vi "Initialize.vi"(7 "Release all channels first":bool=TRUE, 8 "error in (no error)":errorcluster, 9 "TPCANBaudrate":T1, 10 "Channel(1~6)":u8=1, 11 "PCANUSB in":refnum<class "PCANUSB.lvclass">) -> (0 "error out":errorcluster, 3 "PCANUSB out":refnum<class "PCANUSB.lvclass">)   [LabVIEW 2024, in "PCANUSB.lvclass"]
uses:
  PCANUSB.lvclass
  PCAN/CAN Communication.llb/TPCANBaudrate.ctl
  PCAN/CAN Communication.llb/TPCANParameter.ctl
  PCAN/API_for_PCAN_BASIC_FD/TPCANHandle.ctl
  PCANUSB.lvclass/PCANUSB.ctl
  PCAN/CAN Communication.llb/PCAN Get CHANNEL CONDITION.vi
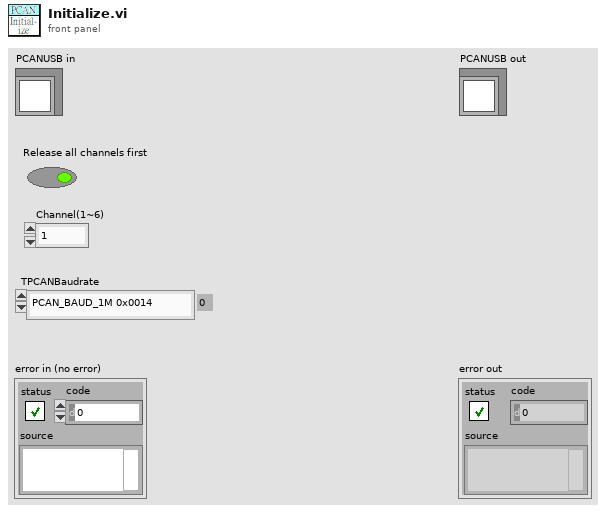
[diagram p1: front panel]
types:
  T1 = typedef "TPCANBaudrate.ctl" = enum16{"PCAN_BAUD_1M 0x0014", "PCAN_BAUD_800K 0x0016", "PCAN_BAUD_500K 0x001C", "PCAN_BAUD_250K 0x011C", "PCAN_BAUD_125K 0x031C", "PCAN_BAUD_100K 0x432F", "PCAN_BAUD_95K 0xC34E", "PCAN_BAUD_83K 0x852B", "PCAN_BAUD_50K 0x472F", "PCAN_BAUD_47K 0x1414", "PCAN_BAUD_33K 0x8B2F", "PCAN_BAUD_20K 0x532F", "PCAN_BAUD_10K 0x672F", "PCAN_BAUD_5K 0x7F7F", "User Baudrate"}
  T2 = typedef "TPCANParameter.ctl" = enum8{"Not Available", "PCAN device number", "PCAN 5-volt power", "PCAN receive event", "PCAN message filter", "PCAN API version", "PCAN channel version", "PCAN busoff autoreset", "PCAN listen-only", "PCAN log location", "PCAN log status", "PCAN log configure", "PCAN log text", "PCAN channel condition", "PCAN hardware name", "PCAN_RECEIVE_STATUS", "PCAN_CONTROLLER_NUMBER", "PCAN_TRACE_LOCATION ", "PCAN_TRACE_STATUS", "PCAN_TRACE_SIZE", "PCAN_TRACE_CONFIGURE", "PCAN_CHANNEL_IDENTIFYING", "PCAN_CHANNEL_FEATURES", "PCAN_SPEED_ADAPTING", "PCAN_BITRATE_INFO", "PCAN_BITRATE_INFO_FD", "PCAN_BUSSPEED_NOMINAL", "PCAN_BUSSPEED_DATA", "PCAN_IP_ADDRESS", "PCAN_LAN_SERVICE_STATUS", "PCAN_ALLOW_STATUS_FRAMES", "PCAN_ALLOW_RTR_FRAMES", "PCAN_ALLOW_ERROR_FRAMES", "PCAN_INTERFRAME_DELAY", "PCAN_ACCEPTANCE_FILTER_11BIT", "PCAN_ACCEPTANCE_FILTER_29BIT", "PCAN_IO_DIGITAL_CONFIGURATION", "PCAN_IO_DIGITAL_VALUE", "PCAN_IO_DIGITAL_SET", "PCAN_IO_DIGITAL_CLEAR", "PCAN_IO_ANALOG_VALUE"}
  T3 = typedef "TPCANHandle.ctl" = enum16{"PCAN_NONEBUS  0x000", "PCAN_ISABUS1  0x21", "PCAN_ISABUS2  0x22", "PCAN_ISABUS3  0x23", "PCAN_ISABUS4  0x24", "PCAN_ISABUS5  0x25", "PCAN_ISABUS6  0x26", "PCAN_ISABUS7  0x27", "PCAN_ISABUS8  0x28", "PCAN_DNGBUS1  0x31", "PCAN_PCIBUS1  0x41", "PCAN_PCIBUS1  0x42", "PCAN_PCIBUS1  0x43", "PCAN_PCIBUS1  0x44", "PCAN_PCIBUS1  0x45", "PCAN_PCIBUS1  0x46", "PCAN_PCIBUS1  0x47", "PCAN_PCIBUS1  0x48", "PCAN_PCIBUS1  0x409", "PCAN_PCIBUS1  0x40A", "PCAN_PCIBUS1  0x40B", "PCAN_PCIBUS1  0x40C", "PCAN_PCIBUS1  0x40D", "PCAN_PCIBUS1  0x40E", "PCAN_PCIBUS1  0x40F", "PCAN_PCIBUS1  0x410", "PCAN_USBBUS1  0x51", "PCAN_USBBUS2  0x52", "PCAN_USBBUS3  0x53", "PCAN_USBBUS4  0x54", "PCAN_USBBUS5  0x55", "PCAN_USBBUS6  0x56", "PCAN_USBBUS7  0x57", "PCAN_USBBUS8  0x58", "PCAN_USBBUS9  0x509", "PCAN_USBBUS10  0x50A", "PCAN_USBBUS11  0x50B", "PCAN_USBBUS12  0x50C", "PCAN_USBBUS13  0x50D", "PCAN_USBBUS14  0x50E", "PCAN_USBBUS15  0x50F", "PCAN_USBBUS16  0x510", "PCAN_PCCBUS1  0x61", "PCAN_PCCBUS2  0x62", "PCAN_LANBUS1  0x801", "PCAN_LANBUS2  0x802", "PCAN_LANBUS3  0x803", "PCAN_LANBUS4  0x804", "PCAN_LANBUS5  0x805", "PCAN_LANBUS6  0x806", "PCAN_LANBUS7  0x807", "PCAN_LANBUS8  0x808", "PCAN_LANBUS9  0x809", "PCAN_LANBUS10  0x80A", "PCAN_LANBUS11  0x80B", "PCAN_LANBUS12  0x80C", "PCAN_LANBUS13  0x80D", "PCAN_LANBUS14  0x80E", "PCAN_LANBUS15  0x80F", "PCAN_LANBUS16  0x810"}
  T4 = typedef "Channel Availability.ctl" = enum16{"PCAN_CHANNEL_UNAVAILABLE", "PCAN_CHANNEL_AVAILABLE", "PCAN_CHANNEL_OCCUPIED"}
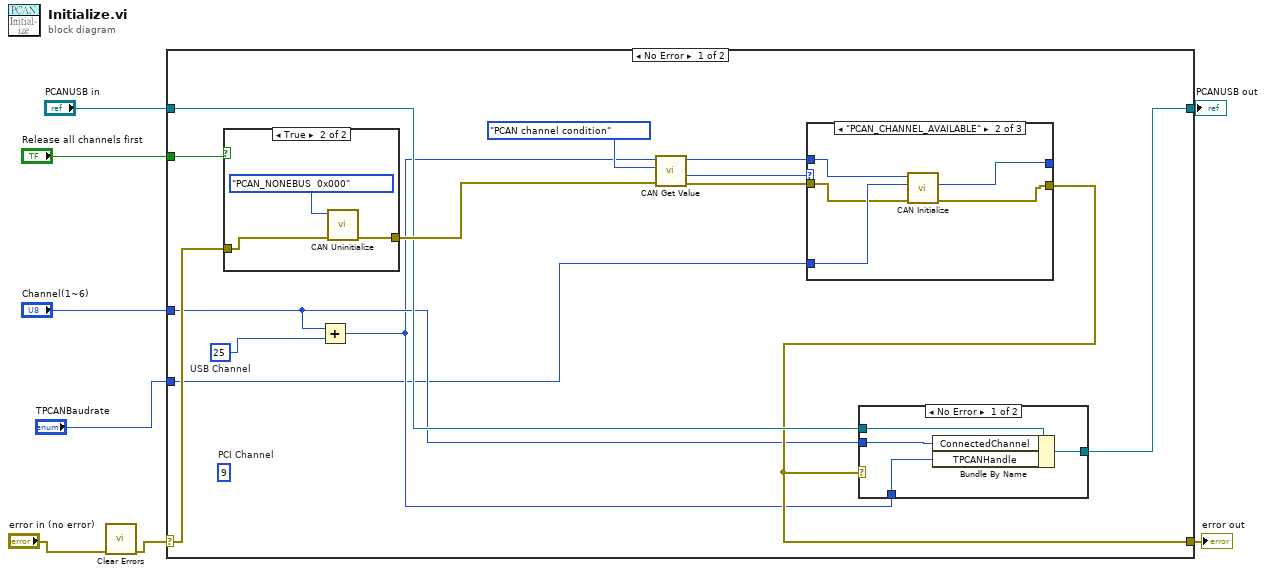
[diagram p0: block diagram]
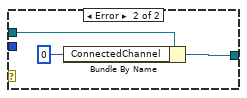
[diagram p2: hidden frame]
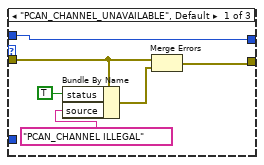
[diagram p3: hidden frame]
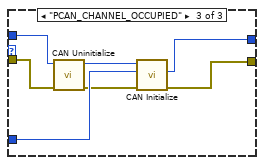
[diagram p4: hidden frame]
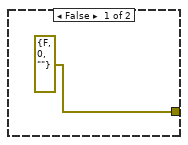
[diagram p5: hidden frame]
diagram:
  n1 = call <vilib>:"Clear Errors.vi"("error in (no error)"="error in (no error)") -> ("error out"=w1:errorcluster)  [unwired: 5 in, 1 out]
  n2 = case shown="No Error" w1 {
    selector: w1 -> [w21 w53]
    tunnel: [w13 w53] -> w8
    tunnel: [w14 w52] -> w6
    tunnel: "PCANUSB in" -> [w15 w52]
    tunnel: "Release all channels first" -> [w22 _]
    tunnel: "TPCANBaudrate" -> [w10 _]
    tunnel: "Channel(1~6)" -> [w12 _]
    frame No Error {
      w9 = 25  # USB Channel
      (unwired) 9  # PCI Channel
      n3 = case shown="True" w22 {
        tunnel: w21 -> [_ w50]
        tunnel: [errorcluster {"status"=FALSE, "code"=0, "source"=""} ("error constant") w49] -> w19
        frame False {
        }
        frame True {
          n4 = call "CAN Uninitialize.vi"("error in (no error)"=w50, "TPCANHandle"=TPCANHandle."PCAN_NONEBUS  0x000") -> ("error out"=w49:errorcluster)  [unwired: 7 in, 2 out]
        }
      }
      n5 = Add(x=w12, y=w9) -> (x+y=w11:i32)
      n6 = call-poly "CAN Get Value.vi"("error in (no error)"=w19, "TPCANParameter"=TPCANParameter."PCAN channel condition", "TPCANHandle"=w11) -> ("error out"=w17:errorcluster, "Channel condition"=w18:T4, "TPCANHandle out"=w16:T3)  [unwired: 6 in]
      n7 = case shown="\"PCAN_CHANNEL_AVAILABLE\"" w18 {
        tunnel: w17 -> [w33 w36 w47]
        tunnel: [w31 w37 w41] -> w13
        tunnel: w16 -> [w30 w40 w46]
        tunnel: w10 -> [_ w39 w44]
        tunnel: [w30 w38 w42] -> _
        frame "PCAN_CHANNEL_UNAVAILABLE", Default {
          n8 = Bundle By Name(cluster=w33, "status"=TRUE, "source"="PCAN_CHANNEL ILLEGAL") -> (w32:errorcluster)
          n9 = Merge Errors(w33, w32) -> (w31:errorcluster)
        }
        frame "PCAN_CHANNEL_AVAILABLE" {
          n10 = call "CAN Initialize.vi"("error in (no error)"=w36, "TPCANBaudrate"=w39, "TPCANHandle"=w40) -> ("error out"=w37:errorcluster, "TPCANHandle_out"=w38:T3)  [unwired: 6 in, 1 out]
        }
        frame "PCAN_CHANNEL_OCCUPIED" {
          n11 = call "CAN Uninitialize.vi"("error in (no error)"=w47, "TPCANHandle"=w46) -> ("error out"=w43:errorcluster, "TPCANHandle out"=w45:T3)  [unwired: 7 in, 1 out]
          n12 = call "CAN Initialize.vi"("error in (no error)"=w43, "TPCANBaudrate"=w44, "TPCANHandle"=w45) -> ("error out"=w41:errorcluster, "TPCANHandle_out"=w42:T3)  [unwired: 6 in, 1 out]
        }
      }
      n13 = case shown="No Error" w13 {
        tunnel: w15 -> [w26 w29]
        tunnel: w12 -> [w25 _]
        tunnel: [w24 w28] -> w14
        tunnel: w11 -> [w23 _]
        frame No Error {
          n14 = Bundle By Name(cluster=w26, "ConnectedChannel"=w25, "TPCANHandle"=w23) -> (w24:refnum<class "PCANUSB.lvclass">)
        }
        frame Error {
          n15 = Bundle By Name(cluster=w29, "ConnectedChannel"=u8 0) -> (w28:refnum<class "PCANUSB.lvclass">)
        }
      }
    }
    frame Error {
    }
  }
  "error out" <- w8
  "PCANUSB out" <- w6
